vi "Erase and Write pulse control V2.0.vi"(8 "error in":errorcluster, 11 "Pulse Settings":T2={"Set point"=-0.03, "Set Resistance"=enum."0 ohms", "First pulse voltage"=0.0, "First pulse time"=10, "Wait between"=0, "Second pulse voltage"=0.0, "Second pulse time"=500, "Withdraw tip? 1"=FALSE, "Set Resistance 2"=enum."0 ohms", "Withdraw tip? 2"=TRUE} {"Second pulse voltage" format="%_5p"; "First pulse voltage" format="%_5p"; "Set point" format="%#_6p"}) -> (0 "error out":errorcluster)   [LabVIEW 2016]
uses:
  <userlib>/LevyLab/Relay Box/Type_defs/Resistor--enum.ctl
panel:
  out "error out 2":errorcluster
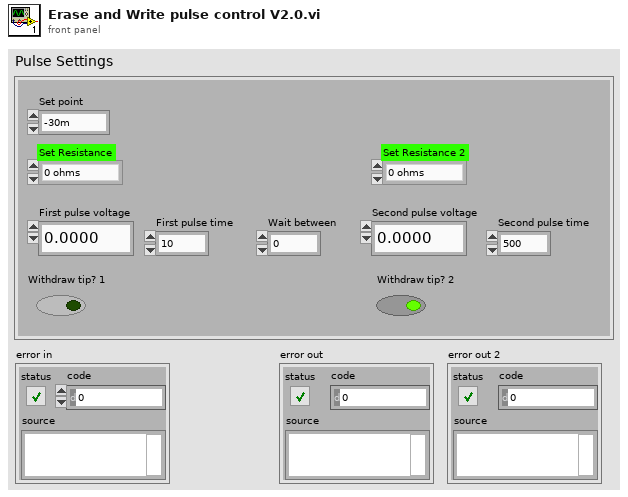
[diagram p1: front panel]
types:
  T1 = typedef "Resistor--enum.ctl" = enum16{"open", "discharge tip", "0 ohms", "100k ohm", "10M ohm", "1G ohm"}
  T2 = cluster{"Set point":dbl, "Set Resistance":T1, "First pulse voltage":dbl, "First pulse time":u32, "Wait between":u32, "Second pulse voltage":dbl, "Second pulse time":u32, "Withdraw tip? 1":bool, "Set Resistance 2":T1, "Withdraw tip? 2":bool}
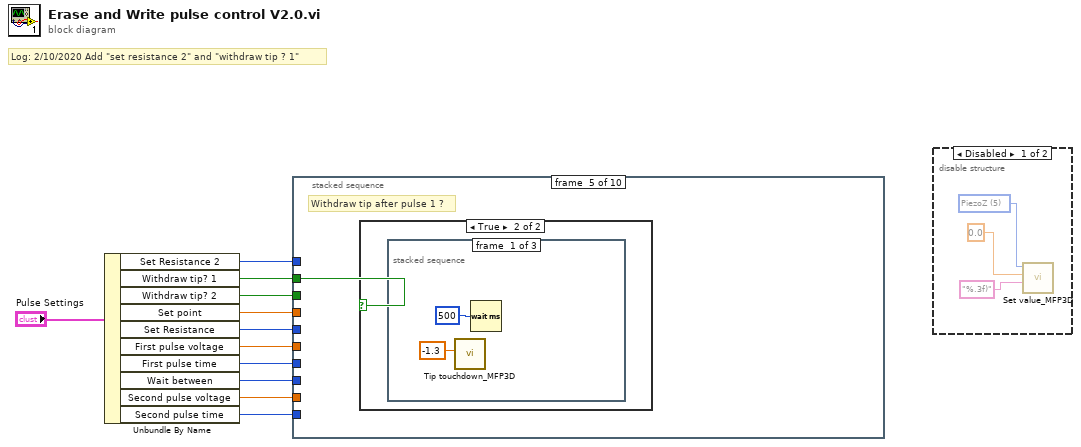
[diagram p0: block diagram]
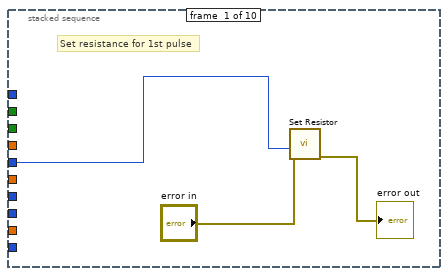
[diagram p3: hidden frame]
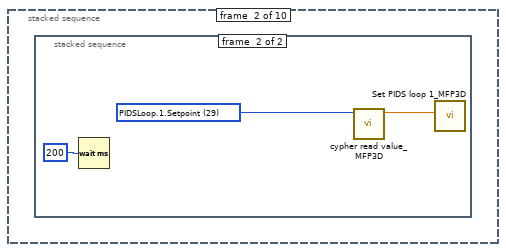
[diagram p4: hidden frame]
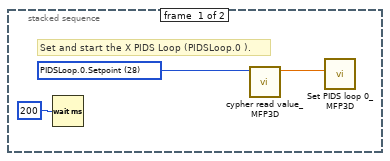
[diagram p5: hidden frame]
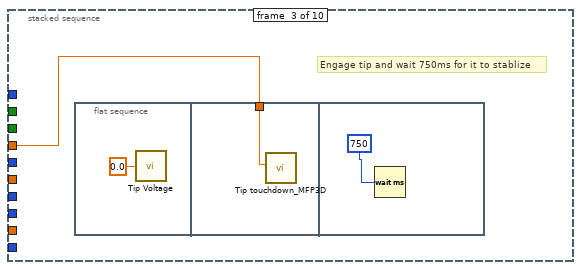
[diagram p6: hidden frame]
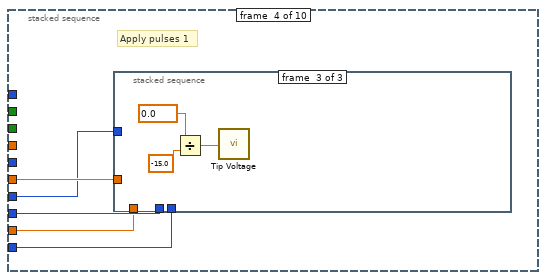
[diagram p7: hidden frame]
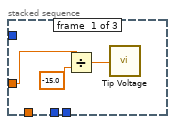
[diagram p8: hidden frame]
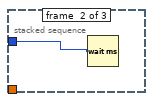
[diagram p9: hidden frame]
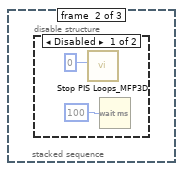
[diagram p11: hidden frame]
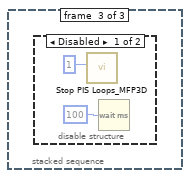
[diagram p13: hidden frame]
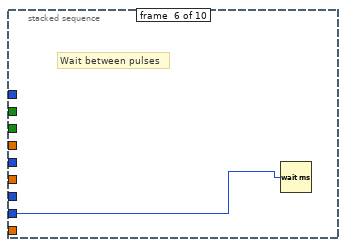
[diagram p15: hidden frame]
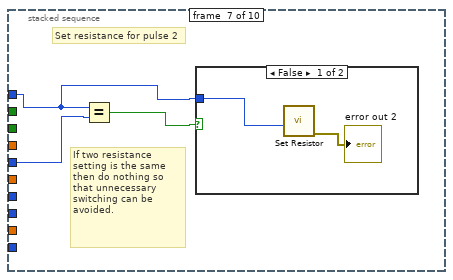
[diagram p16: hidden frame]
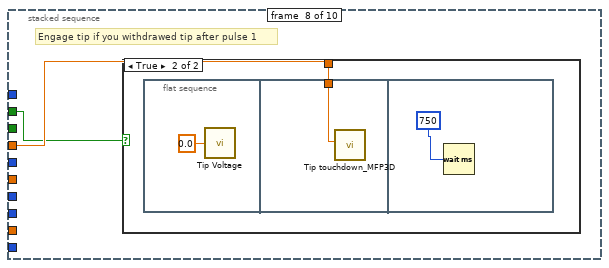
[diagram p18: hidden frame]
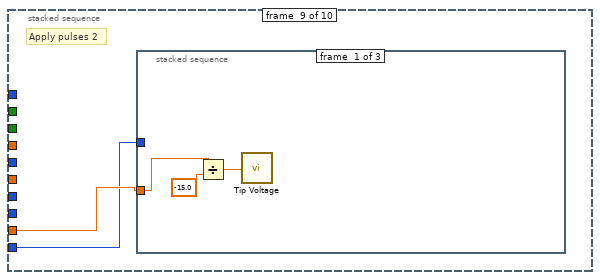
[diagram p20: hidden frame]
diagram:
  # "Log: 2/10/2020 Add \"set resistance 2\" and \"withdraw tip ? 1\""
  n1 = Unbundle By Name("Pulse Settings") -> ("Set Resistance 2"=w1:T1, "Withdraw tip? 1"=w2:bool, "Withdraw tip? 2"=w3:bool, "Set point"=w9:dbl, "Set Resistance"=w10:T1, "First pulse voltage"=w8:dbl, "First pulse time"=w7:u32, "Wait between"=w6:u32, "Second pulse voltage"=w5:dbl, "Second pulse time"=w4:u32)
  n2 = stacked-sequence {
    tunnel: w10 -> [w12 _ _ _ _ _ w47 _ _ _]
    tunnel: w9 -> [_ _ w21 _ _ _ _ w51 _ w66]
    tunnel: w8 -> [_ _ _ w29 _ _ _ _ _ _]
    tunnel: w7 -> [_ _ _ w28 _ _ _ _ _ _]
    tunnel: w6 -> [_ _ _ w27 _ w44 _ _ _ _]
    tunnel: w5 -> [_ _ _ w26 _ _ _ _ w57 _]
    tunnel: w4 -> [_ _ _ w25 _ _ _ _ w56 _]
    tunnel: w3 -> [_ _ _ _ _ _ _ _ _ w65]
    tunnel: w2 -> [_ _ _ _ w37 _ _ w50 _ _]
    tunnel: w1 -> [_ _ _ _ _ _ w45 _ _ _]
    frame #0 {
      # "Set resistance for 1st pulse"
      n3 = call <userlib>:"Set Resistor.vi"("error in"="error in", "Set Resistance"=w12) -> ("error out"=→"error out":errorcluster)  [unwired: 9 in]
    }
    frame #1 {
      n4 = stacked-sequence {
        frame #0 {
          w16 = u16 28 items=["XSensor", "YSensor", "ZSensor", "InA", "InB", "InFast", "In_Amplitude1", "In_Amplitude2", "In_Phase1", "In_Phase2", "PiezoX", "PiezoY", "PiezoZ", "OutA", "OutB", "OutC", "DDS_Frequency1", "DDS_Frequency2", "DDS_Amplitude1", "DDS_Amplitude2", "DDS_DCOffset", "Laser_Sum", "Laser_Difference", "Laser_Lateral", "XLVDT Sensitivity", "YLVDT Sensitivity", "XLVDT Offset", "YLVDT Offset", "PIDSLoop.0.Setpoint", "PIDSLoop.1.Setpoint"] ("Input")
          # "Set and start the X PIDS Loop (PIDSLoop.0 )."
          n5 = Wait (ms)(milliseconds to wait=u32 200) -> ()  [unwired: 1 out]
          n6 = call <userlib>:"cypher read value_MFP3D.vi"("Input"=w16) -> ("Result"=w17:dbl)  [unwired: 10 in]
          n7 = call <userlib>:"Set PIDS loop 0_MFP3D.vi"("X  Setpoint"=w17) -> ()  [unwired: 11 in]
        }
        frame #1 {
          w19 = u16 29 items=["XSensor", "YSensor", "ZSensor", "InA", "InB", "InFast", "In_Amplitude1", "In_Amplitude2", "In_Phase1", "In_Phase2", "PiezoX", "PiezoY", "PiezoZ", "OutA", "OutB", "OutC", "DDS_Frequency1", "DDS_Frequency2", "DDS_Amplitude1", "DDS_Amplitude2", "DDS_DCOffset", "Laser_Sum", "Laser_Difference", "Laser_Lateral", "XLVDT Sensitivity", "YLVDT Sensitivity", "XLVDT Offset", "YLVDT Offset", "PIDSLoop.0.Setpoint", "PIDSLoop.1.Setpoint"] ("Input")
          n8 = Wait (ms)(milliseconds to wait=u32 200) -> ()  [unwired: 1 out]
          n9 = call <userlib>:"cypher read value_MFP3D.vi"("Input"=w19) -> ("Result"=w18:dbl)  [unwired: 10 in]
          n10 = call <userlib>:"Set PIDS loop 1_MFP3D.vi"("Y Setpoint"=w18) -> ()  [unwired: 11 in]
        }
      }
    }
    frame #2 {
      # "Engage tip and wait 750ms for it to stablize"
      n11 = flat-sequence {
        tunnel: w21 -> [w23]
        frame #0 {
          n12 = call <userlib>:"Tip Voltage.vi"("Output Voltage"=0.0) -> ()  [unwired: 1 out]
        }
        frame #1 {
          n13 = call <userlib>:"Tip touchdown_MFP3D.vi"("Z SetPoint"=w23) -> ()  [unwired: 11 out]
        }
        frame #2 {
          n14 = Wait (ms)(milliseconds to wait=u32 750 ("Wait time first pulse  2")) -> ()  [unwired: 1 out]
        }
      }
    }
    frame #3 {
      # "Apply pulses 1"
      n15 = stacked-sequence {
        tunnel: w29 -> [w30 _ _]
        tunnel: w28 -> [_ w33 _]
        tunnel: w27 -> [_ _ _]
        tunnel: w26 -> [_ _ _]
        tunnel: w25 -> [_ _ _]
        frame #0 {
          n16 = Divide(x=w30, y=-15.0) -> (x/y=w31:dbl)
          n17 = call <userlib>:"Tip Voltage.vi"("Output Voltage"=w31) -> ()  [unwired: 1 out]
        }
        frame #1 {
          n18 = Wait (ms)(milliseconds to wait=w33) -> ()  [unwired: 1 out]
        }
        frame #2 {
          n19 = Divide(x=0.0 ("Output Voltage 2"), y=-15.0) -> (x/y=w36:dbl)
          n20 = call <userlib>:"Tip Voltage.vi"("Output Voltage"=w36) -> ()  [unwired: 1 out]
        }
      }
    }
    frame #4 {
      # "Withdraw tip after pulse 1 ?"
      n21 = case shown="True" w37 {
        frame False {
        }
        frame True {
          n22 = stacked-sequence {
            frame #0 {
              n23 = call <userlib>:"Tip touchdown_MFP3D.vi"("Z SetPoint"=-1.3) -> ()  [unwired: 11 out]
              n24 = Wait (ms)(milliseconds to wait=u32 500) -> ()  [unwired: 1 out]
            }
            frame #1 {
              n25 = disable-structure shown="Disabled" {
                frame Disabled {
                  n26 = call <userlib>:"Stop PIS Loops_MFP3D.vi"("PIS Loop Number (0-5)"=u32 0) -> ()  [unwired: 11 out]
                  n27 = Wait (ms)(milliseconds to wait=u32 100) -> ()  [unwired: 1 out]
                }
                frame Enabled {
                }
              }
            }
            frame #2 {
              n28 = disable-structure shown="Disabled" {
                frame Disabled {
                  n29 = call <userlib>:"Stop PIS Loops_MFP3D.vi"("PIS Loop Number (0-5)"=u32 1) -> ()  [unwired: 11 out]
                  n30 = Wait (ms)(milliseconds to wait=u32 100) -> ()  [unwired: 1 out]
                }
                frame Enabled {
                }
              }
            }
          }
        }
      }
    }
    frame #5 {
      # "Wait between pulses"
      n31 = Wait (ms)(milliseconds to wait=w44) -> ()  [unwired: 1 out]
    }
    frame #6 {
      # "Set resistance for pulse 2"
      # "If two resistance setting is the same then do nothing so that unnecessary switching can be avoided."
      n32 = Equal?(x=w45, y=w47) -> (x = y?=w46:bool)
      n33 = case shown="False" w46 {
        tunnel: w45 -> [w49 _]
        frame False {
          n34 = call <userlib>:"Set Resistor.vi"("Set Resistance"=w49) -> ("error out"=→"error out 2":errorcluster)  [unwired: 10 in]
        }
        frame True {
        }
      }
    }
    frame #7 {
      # "Engage tip if you withdrawed tip after pulse 1"
      n35 = case shown="True" w50 {
        tunnel: w51 -> [_ w52]
        frame False {
        }
        frame True {
          n36 = flat-sequence {
            tunnel: w52 -> [w54]
            frame #0 {
              n37 = call <userlib>:"Tip Voltage.vi"("Output Voltage"=0.0) -> ()  [unwired: 1 out]
            }
            frame #1 {
              n38 = call <userlib>:"Tip touchdown_MFP3D.vi"("Z SetPoint"=w54) -> ()  [unwired: 11 out]
            }
            frame #2 {
              n39 = Wait (ms)(milliseconds to wait=u32 750 ("Wait time first pulse  2")) -> ()  [unwired: 1 out]
            }
          }
        }
      }
    }
    frame #8 {
      # "Apply pulses 2"
      n40 = stacked-sequence {
        tunnel: w57 -> [w58 _ _]
        tunnel: w56 -> [_ w61 _]
        frame #0 {
          n41 = Divide(x=w58, y=-15.0) -> (x/y=w59:dbl)
          n42 = call <userlib>:"Tip Voltage.vi"("Output Voltage"=w59) -> ()  [unwired: 1 out]
        }
        frame #1 {
          n43 = Wait (ms)(milliseconds to wait=w61) -> ()  [unwired: 1 out]
        }
        frame #2 {
          n44 = Divide(x=0.0 ("Output Voltage 2"), y=-15.0) -> (x/y=w64:dbl)
          n45 = call <userlib>:"Tip Voltage.vi"("Output Voltage"=w64) -> ()  [unwired: 1 out]
        }
      }
    }
    frame #9 {
      # "Withdraw tip after pulse 2 ?"
      n46 = case shown="True" w65 {
        tunnel: w66 -> [w67 _]
        frame False {
          # "Maybe I can empty this case"
          n47 = disable-structure shown="Disabled" {
            disable-tunnel: w67 -> [w68 _]
            frame Disabled {
              n48 = call <userlib>:"Tip touchdown_MFP3D.vi"("Z SetPoint"=w68) -> ()  [unwired: 11 out]
            }
            frame Enabled {
            }
          }
        }
        frame True {
          n49 = stacked-sequence {
            frame #0 {
              n50 = disable-structure shown="Disabled" {
                frame Disabled {
                  n51 = call <userlib>:"Tip Withdraw_MFP3D.vi"() -> ()  [unwired: 1 in]
                }
                frame Enabled {
                }
              }
              n52 = call <userlib>:"Tip touchdown_MFP3D.vi"("Z SetPoint"=-1.3) -> ()  [unwired: 11 out]
              n53 = Wait (ms)(milliseconds to wait=u32 500) -> ()  [unwired: 1 out]
            }
            frame #1 {
              n54 = disable-structure shown="Disabled" {
                frame Disabled {
                  n55 = call <userlib>:"Stop PIS Loops_MFP3D.vi"("PIS Loop Number (0-5)"=u32 0) -> ()  [unwired: 11 out]
                  n56 = Wait (ms)(milliseconds to wait=u32 100) -> ()  [unwired: 1 out]
                }
                frame Enabled {
                }
              }
            }
            frame #2 {
              n57 = disable-structure shown="Disabled" {
                frame Disabled {
                  n58 = call <userlib>:"Stop PIS Loops_MFP3D.vi"("PIS Loop Number (0-5)"=u32 1) -> ()  [unwired: 11 out]
                  n59 = Wait (ms)(milliseconds to wait=u32 100) -> ()  [unwired: 1 out]
                }
                frame Enabled {
                }
              }
            }
          }
        }
      }
    }
  }
  n60 = disable-structure shown="Disabled" {
    frame Disabled {
      w77 = u16 5 items=["OutA_52kHz", "OutB_52kHz", "OutC_78Hz", "PiezoX", "PiezoY", "PiezoZ", "DDS_Frequency1", "DDS_Frequency2", "DDS_Amplitude1", "DDS_Amplitude2"] ("Output")
      n61 = call <userlib>:"Set value_MFP3D.vi"("Number resolutio"="%.3f)", "Value"=0.0, "Output"=w77) -> ()  [unwired: 8 in, 1 out]
    }
    frame Enabled {
    }
  }
